vi "set_column_readonly.vi"(8 "error in (no error)":errorcluster, 9 "ReadOnly?":bool=TRUE, 10 "Col_idx":u32, 11 "DataTable In":refnum<class "DataTable.lvclass">) -> (0 "error out":errorcluster, 3 "DataTable Out":refnum<class "DataTable.lvclass">)   [LabVIEW 2015, in "DataGrid.lvlib" / "DataTable.lvclass"]
uses:
  DataTable.lvclass
  DataTable.lvclass/DataTable.ctl
  System.Data
  Read DataTable.vi
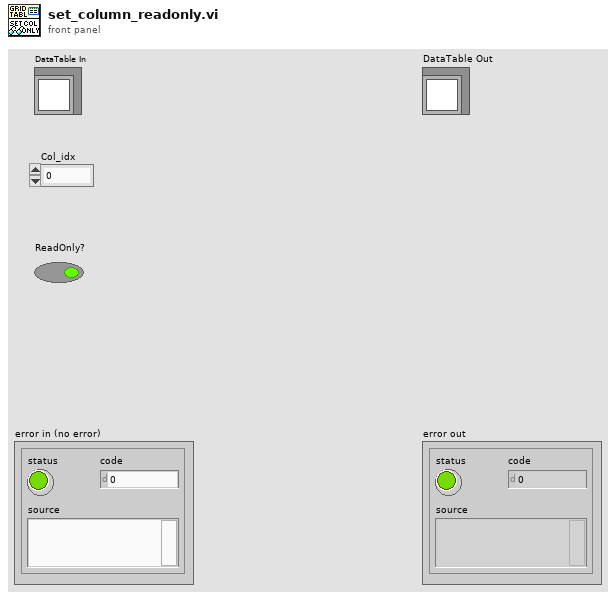
[diagram p1: front panel]
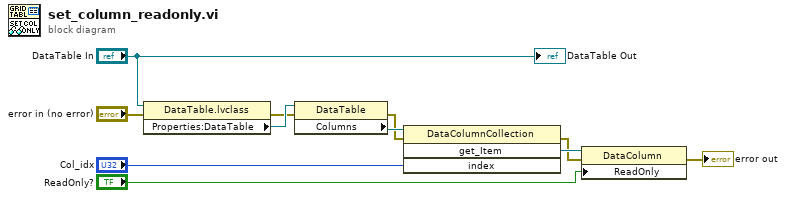
[diagram p0: block diagram]
diagram:
  n1 = property class="DataTable.lvclass"(reference="DataTable In", error in="error in (no error)") -> (error out=w9:errorcluster, "Properties:DataTable"=w11:refnum<k24>)  [unwired: 1 out]
  n2 = property class="DataTable"(reference=w11, error in=w9) -> (error out=w2:errorcluster, "Columns"=w7:refnum<k24>)  [unwired: 1 out]
  n3 = invoke class="DataColumnCollection" method="get_Item"(reference=w7, error in=w2, "index"="Col_idx") -> (error out=w3:errorcluster, "get_Item"=w6:refnum<k24>)  [unwired: 1 in, 2 out]
  n4 = property class="DataColumn"(reference=w6, error in=w3, "ReadOnly"="ReadOnly?") -> (error out=→"error out":errorcluster)  [unwired: 1 out]
  "DataTable Out" <- "DataTable In"
